vi "ScpGetPreSampleRatio.vi"(0 "hDevice in":u32, 3 "error in (no error)":errorcluster) -> (7 "hDevice out":u32, 8 "dPreSampleRatio":dbl, 10 "error out":errorcluster)   [LabVIEW 2018, in "LibTiePie.lvlib"]
uses:
  LibTiePie.lvlib
  LabViewHS4/libtiepie.dll
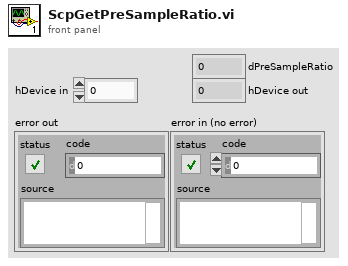
[diagram p1: front panel]
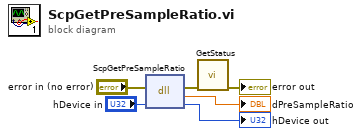
[diagram p0: block diagram]
diagram:
  n1 = dll-call lib="C:/Users/cwaha/Documents/LabViewHS4/libtiepie.dll" fn="ScpGetPreSampleRatio"(error in="error in (no error)", "hDevice"="hDevice in") -> (error out=w6:errorcluster, "dPreSampleRatio"=→"dPreSampleRatio":dbl, "hDevice"=→"hDevice out":u32)  [unwired: 2 in, 1 out]
  n2 = call "GetStatus.vi"("error in (no error)"=w6) -> ("error out"=→"error out":errorcluster)  [unwired: 10 in]
